vi "Set Trigger.vi"(8 "error in (no error)":errorcluster, 11 "CCDCamera in":refnum<class "CCDCamera.lvclass">) -> (0 "error out":errorcluster, 3 "CCDCamera out":refnum<class "CCDCamera.lvclass">)   [LabVIEW 2018, in "CCDCamera.lvclass"]
uses:
  CCDCamera.lvclass
  C:/Users/observer/Desktop/SPARC4_ACS/SPARC4_ACS/Simulated_CCD_Camera/Simulated_CCD_Camera.lvclass
  Simulated_CCD_Camera/Simulated_CCD_Camera.lvclass/Simulated_CCD_Camera.ctl
  Interface/Interface.lvclass
  Simulated_CCD_Camera/Simulated_CCD_Camera.lvclass
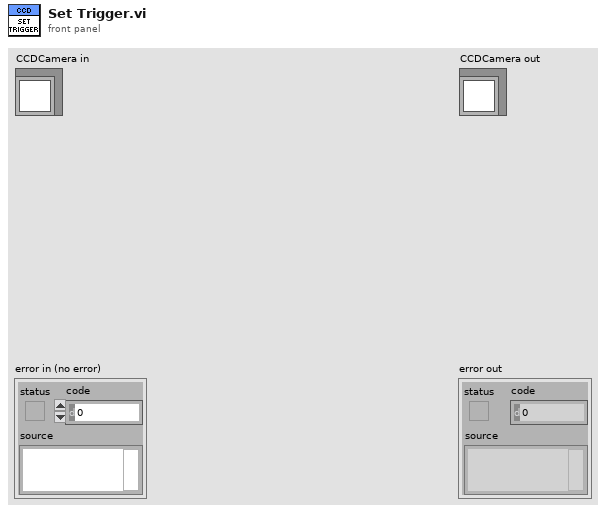
[diagram p1: front panel]
types:
  T1 = typedef "Shutter_mode typedef.ctl" = enum16{"Auto", "Open", "Close", "N/A (3)", "Open FVB Series", "Open Any Series"}
  T2 = typedef "ReadMode_mode typedef.ctl" = enum16{"Full Vertical Binning", "Multi-Track", "Random-Track", "Single-Track", "Image"}
  T3 = typedef "AcquisitionMode_mode typedef.ctl" = enum16{"Reserved (0)", "Single Scan", "Accumulate", "Kinetics", "Fast Kinetics", "Run Till Abort", "Reserved (6)", "Reserved (7)", "Reserved (8)", "Time Delayed Integration"}
  T4 = cluster{"PREAMP":enum16{"Gain 1", "Gain 2"}, "READOUT_RATE":enum16{"30 MHz", "20 MHz", "10 MHz", "1 MHz"}, "EM_GAIN":u16, "VBIN":u16, "INITIAL_LINE":u16, "INITIAL_COLUMN":u16, "FINAL_LINE":u16, "FINAL_COLUMN":u16, "TRIGGER_MODE":enum16{"Internal", "External", "N/A", "N/A_1", "N/A_2", "N/A_3", "External Start"}, "HBIN":u16, "SHUTTER_TTL":enum16{"TTL Low", "TTL High"}, "SHUTTER_MODE":T1, "SHUTTER_OPENING_TIME":u16, "SHUTTER_CLOSING_TIME":u16, "VERTICAL_SHIFT_SPEED":u16, "READ_MODE":T2, "FRAME_TRANSFER":bool, "VERTICAL_CLOCK_VOLTAGE":enum16{"0", "+1", "+2", "+3", "+4"}, "ACQUISITION_MODE":T3, "AD_CHANNEL":u16, "EM_MODE":enum16{"Electron Multiplying", "Conventional"}}
  T5 = cluster{"PREAMP":u16, "READOUT_RATE":u16, "EM_GAIN":u16, "VBIN":u16, "INITIAL_LINE":u16, "INITIAL_COLUMN":u16, "FINAL_LINE":u16, "FINAL_COLUMN":u16, "TRIGGER_MODE":u16, "HBIN":u16, "SHUTTER_TTL":u16, "SHUTTER_MODE":u16, "SHUTTER_OPENING_TIME":u16, "SHUTTER_CLOSING_TIME":u16, "VERTICAL_SHIFT_SPEED":u16, "READ_MODE":u16, "FRAME_TRANSFER":bool, "VERTICAL_CLOCK_VOLTAGE":u16, "ACQUISITION_MODE":u16, "AD_CHANNEL":u16, "EM_MODE":u16}
  T6 = enum16{"Internal", "External", "N/A", "N/A_1", "N/A_2", "N/A_3", "External Start"}
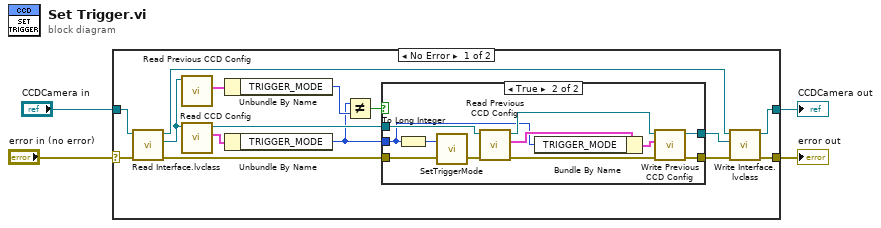
[diagram p0: block diagram]
diagram:
  n1 = case shown="No Error" "error in (no error)" {
    selector: "error in (no error)" -> [w19 w34]
    tunnel: [w8 w34] -> w2
    tunnel: [w6 w33] -> w1
    tunnel: "CCDCamera in" -> [w5 w33]
    frame No Error {
      n2 = call "Read Interface.lvclass.vi"("error in (no error)"=w19, "Simulated_CCD_Camera in"=w5) -> ("error out"=w12:errorcluster, "Interface.lvclass"=w18:refnum<class "Interface.lvclass">, "Simulated_CCD_Camera out"=w9:refnum<class "CCDCamera.lvclass">)  [unwired: 7 in]
      n3 = call "Read Previous CCD Config.vi"("Interface in"=w18) -> ("Previous CCD Config"=w16:T4)  [unwired: 8 in, 2 out]
      n4 = call "Read CCD Config.vi"("Interface in"=w18) -> ("Previous CCD Config"=w17:T5, "Interface out"=w13:refnum<class "Interface.lvclass">)  [unwired: 8 in, 1 out]
      n5 = Unbundle By Name(w16) -> ("TRIGGER_MODE"=w15:T6)
      n6 = Unbundle By Name(w17) -> ("TRIGGER_MODE"=w7:u16)
      n7 = Not Equal?(x=w7, y=w15) -> (x != y?=w14:bool)
      n8 = case shown="True" w14 {
        tunnel: w13 -> [w21 w32]
        tunnel: w12 -> [w20 w24]
        tunnel: [w21 w28] -> w11
        tunnel: [w20 w27] -> w10
        tunnel: w7 -> [_ w22]
        frame False {
        }
        frame True {
          n9 = To Long Integer(number=w22) -> (32bit integer=w23:i32)
          n10 = call <userlib>:"SetTriggerMode.vi"("error in (no error)"=w24, "mode"=w23) -> ("error out"=w25:errorcluster)  [unwired: 1 out]
          n11 = call "Read Previous CCD Config.vi"("error in (no error)"=w25, "Interface in"=w32) -> ("error out"=w26:errorcluster, "Previous CCD Config"=w31:T4, "Interface out"=w29:refnum<class "Interface.lvclass">)  [unwired: 7 in]
          n12 = Bundle By Name(cluster=w31, "TRIGGER_MODE"=w22) -> (w30:T4)
          n13 = call "Write Previous CCD Config.vi"("error in (no error)"=w26, "Previous CCD Config"=w30, "Interface in"=w29) -> ("error out"=w27:errorcluster, "Interface out"=w28:refnum<class "Interface.lvclass">)  [unwired: 7 in]
        }
      }
      n14 = call "Write Interface.lvclass.vi"("error in (no error)"=w10, "Interface.lvclass"=w11, "Simulated_CCD_Camera in"=w9) -> ("error out"=w8:errorcluster, "Simulated_CCD_Camera out"=w6:refnum<class "CCDCamera.lvclass">)  [unwired: 7 in]
    }
    frame Error {
    }
  }
  "error out" <- w2
  "CCDCamera out" <- w1
